vi "RunEcal.vi"(8 "error in (no error)":errorcluster, 11 "NetA_AgNA in":refnum<class "NetA_AgNA.lvclass">) -> (0 "error out":errorcluster {"code" format="%.0x"}, 2 "Error String":string, 3 "NetA_AgNA out":refnum<class "NetA_AgNA.lvclass">)   [LabVIEW 2014, in "NetA_AgNA.lvclass"]
doc: "Commands the eCal to make the specified measurements."
uses:
  NetA_AgNA.lvclass
  Tools/Station Calibration/RFSP MCT Calibration Tool/TypeDefs/TriggerMode_TypeDef.ctl
  Tools/Station Calibration/RFSP MCT Calibration Tool/TypeDefs/TriggerSource_TypeDef.ctl
  NetA_AgNA.lvclass/NetA_AgNA.ctl
  <instrlib>/Agilent NA/Agilent NA.lvlib
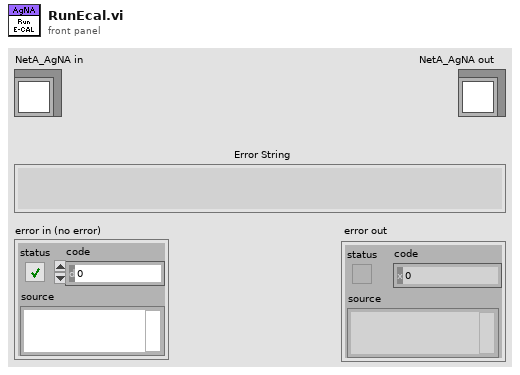
[diagram p1: front panel]
types:
  T1 = typedef "TriggerSource_TypeDef.ctl" = i32
  T2 = typedef "TriggerMode_TypeDef.ctl" = i32
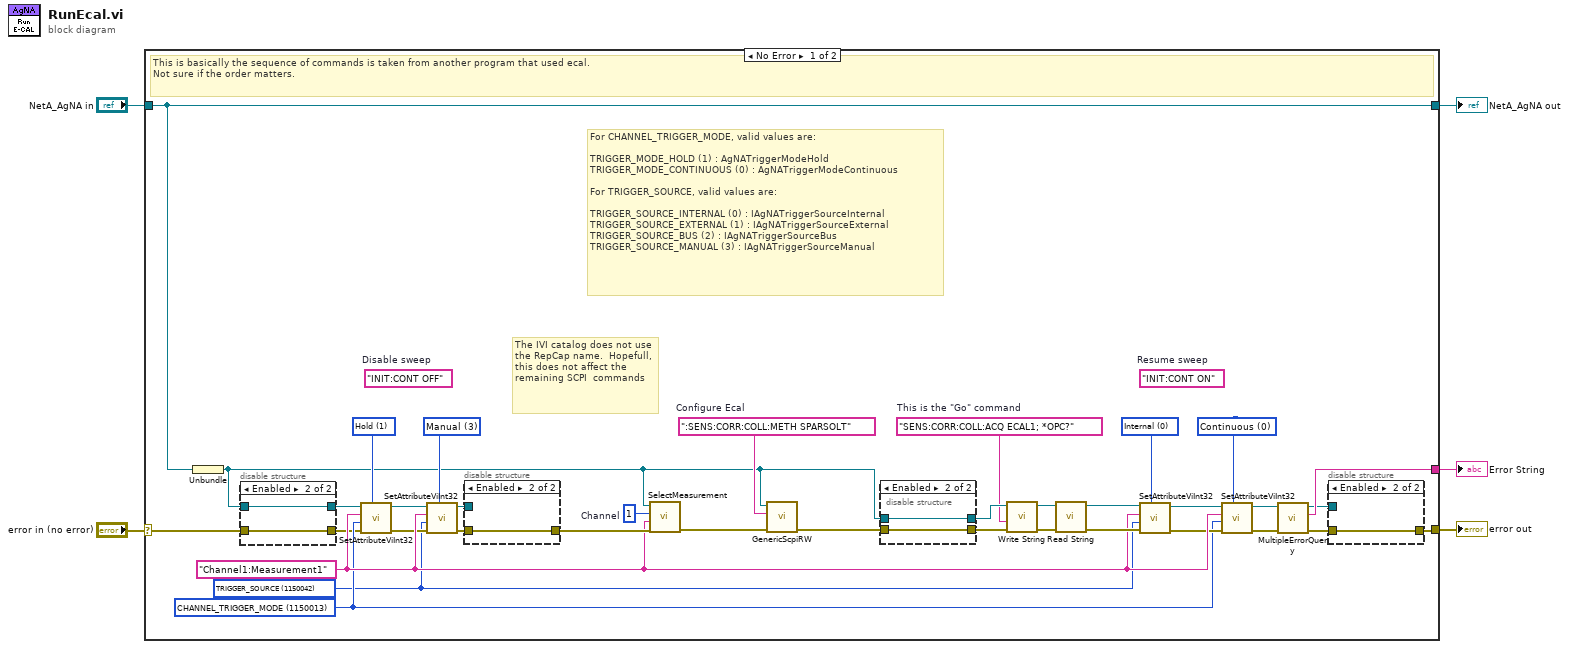
[diagram p0: block diagram]
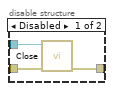
[diagram p2: hidden frame]
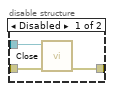
[diagram p3: hidden frame]
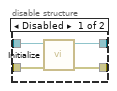
[diagram p4: hidden frame]
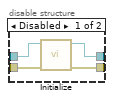
[diagram p5: hidden frame]
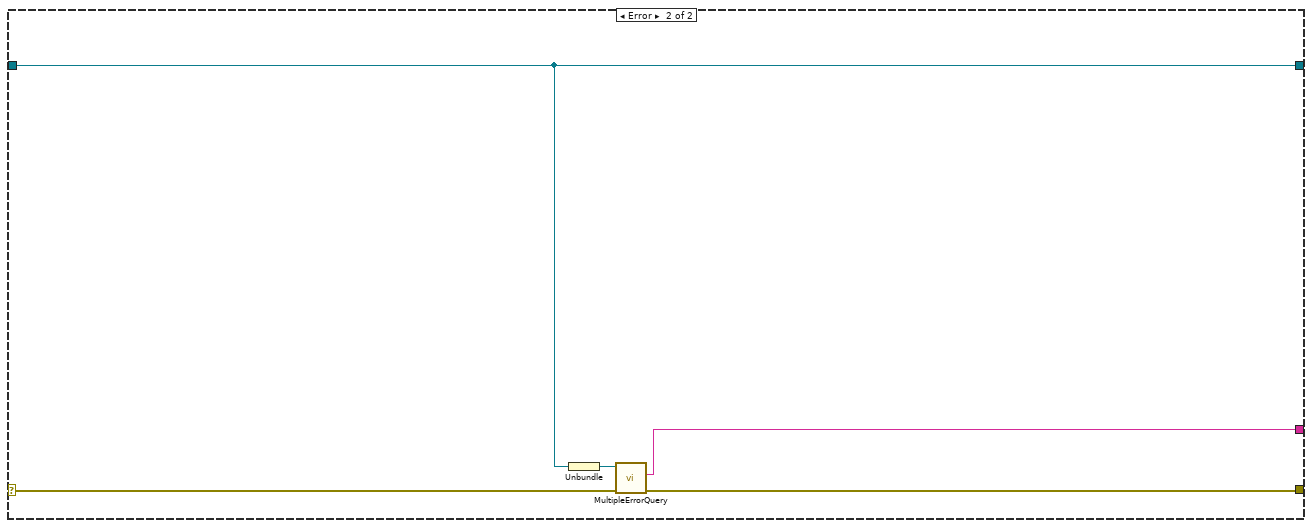
[diagram p6: hidden frame]
diagram:
  n1 = case shown="No Error" "error in (no error)" {
    selector: "error in (no error)" -> [w12 w66]
    tunnel: [w6 w65] -> w4
    tunnel: "NetA_AgNA in" -> [w14 w64]
    tunnel: [w14 w64] -> w2
    tunnel: [w15 w62] -> w1
    frame No Error {
      w13 = u32 1  # Channel
      w16 = T1 0 items=["Internal", "External", "Bus", "Manual"] ("Trigger Source Type")
      w17 = T1 3 items=["Internal", "External", "Bus", "Manual"] ("Trigger Source Type")
      w18 = T2 0 items=["Continuous", "Hold"] ("Trigger Mode Type")
      w19 = T2 1 items=["Continuous", "Hold"] ("Trigger Mode Type")
      (unwired) "INIT:CONT ON"  # Resume sweep
      (unwired) "INIT:CONT OFF"  # Disable sweep
      w23 = u32 1150013 items=["CHANNEL_AVERAGING_FACTOR"=1150002, "CHANNEL_MEASUREMENT_ELECTRICAL_DELAY_MEDIUM"=1150178, "CHANNEL_MEASUREMENT_ELECTRICAL_DELAY_UNITS"=1150175, "CHANNEL_MEASUREMENT_FORMAT"=1150014, "CHANNEL_MEASUREMENT_LIMIT_NUMBER"=1150020, "CHANNEL_MEASUREMENT_TIME_DOMAIN_GATING_SHAPE"=1150140, "CHANNEL_MEASUREMENT_TIME_DOMAIN_GATING_TYPE"=1150144, "CHANNEL_MEASUREMENT_TIME_DOMAIN_PARAMETERS"=1150137, "CHANNEL_MEASUREMENT_TIME_DOMAIN_TRANSFORM_MODE"=1150147, "CHANNEL_MEASUREMENT_TRACE_MATH"=1150017, "CHANNEL_POINTS"=1150007, "CHANNEL_SWEEP_MODE"=1150009, "CHANNEL_SWEEP_TYPE"=1150012, "CHANNEL_TRIGGER_MODE"=1150013, "DISPLAY_ARRANGE_WINDOWS"=1150181, "SYSTEM_TIME_OUT_MILLISECONDS"=1150040, "TRIGGER_SOURCE"=1150042, "WINDOW_SIZE"=1150133, "WINDOW_TABLE"=1150134] ("AttributeID")
      w22 = u32 1150042 items=["CHANNEL_AVERAGING_FACTOR"=1150002, "CHANNEL_MEASUREMENT_ELECTRICAL_DELAY_MEDIUM"=1150178, "CHANNEL_MEASUREMENT_ELECTRICAL_DELAY_UNITS"=1150175, "CHANNEL_MEASUREMENT_FORMAT"=1150014, "CHANNEL_MEASUREMENT_LIMIT_NUMBER"=1150020, "CHANNEL_MEASUREMENT_TIME_DOMAIN_GATING_SHAPE"=1150140, "CHANNEL_MEASUREMENT_TIME_DOMAIN_GATING_TYPE"=1150144, "CHANNEL_MEASUREMENT_TIME_DOMAIN_PARAMETERS"=1150137, "CHANNEL_MEASUREMENT_TIME_DOMAIN_TRANSFORM_MODE"=1150147, "CHANNEL_MEASUREMENT_TRACE_MATH"=1150017, "CHANNEL_POINTS"=1150007, "CHANNEL_SWEEP_MODE"=1150009, "CHANNEL_SWEEP_TYPE"=1150012, "CHANNEL_TRIGGER_MODE"=1150013, "DISPLAY_ARRANGE_WINDOWS"=1150181, "SYSTEM_TIME_OUT_MILLISECONDS"=1150040, "TRIGGER_SOURCE"=1150042, "WINDOW_SIZE"=1150133, "WINDOW_TABLE"=1150134] ("AttributeID")
      w30 = "Channel1:Measurement1" ("Meas Name")
      w36 = "SENS:CORR:COLL:ACQ ECAL1; *OPC?"  # This is the "Go" command
      w41 = ":SENS:CORR:COLL:METH SPARSOLT"  # Configure Ecal
      # "The IVI catalog does not use the RepCap name.  Hopefull, this does not affect the remaining SCPI  commands"
      # "For CHANNEL_TRIGGER_MODE, valid values are:\n\nTRIGGER_MODE_HOLD (1) : AgNATriggerModeHold\nTRIGGER_MODE_CONTINUOUS (0) : AgNATriggerModeContinuous\n\nFor TRIGGER_SOURCE, valid values are:\n\nTRIGGER_SOURCE_INTERNAL (0) : IAgNATriggerSourceInternal  \nTRIGGER_SOURCE_EXTERNAL (1) : IAgNATriggerSourceExternal\nTRIGGER_SOURCE_BUS (2) : IAgNATriggerSourceBus\nTRIGGER_SOURCE_MANUAL (3) : IAgNATriggerSourceManual"
      # "This is basically the sequence of commands is taken from another program that used ecal.\nNot sure if the order matters."
      n2 = Unbundle(w14) -> (w10:refnum<k15>)
      n3 = disable-structure shown="Enabled" {
        disable-tunnel: [w53 w55] -> w11
        disable-tunnel: [w52 w54] -> w9
        disable-tunnel: w12 -> [w51 w55]
        disable-tunnel: w10 -> [w50 w54]
        frame Disabled {
          n4 = call <instrlib>:"Initialize.vi"("error in (no error)"=w51, "resource name"=w50) -> ("error out"=w53:errorcluster, "instrument handle out"=w52:refnum<k15>)  [unwired: 8 in]
        }
        frame Enabled {
        }
      }
      n5 = call <instrlib>:"SetAttributeViInt32.vi"("AttributeValue"=w19, "error in (no error)"=w11, "AttributeID"=w23, "RepCapIdentifier"=w30, "instrument handle"=w9) -> ("error out"=w29:errorcluster, "instrument handle out"=w28:refnum<k15>)  [unwired: 5 in]
      n6 = call <instrlib>:"SetAttributeViInt32.vi"("AttributeValue"=w17, "error in (no error)"=w29, "AttributeID"=w22, "RepCapIdentifier"=w30, "instrument handle"=w28) -> ("error out"=w27:errorcluster, "instrument handle out"=w26:refnum<k15>)  [unwired: 5 in]
      n7 = disable-structure shown="Enabled" {
        disable-tunnel: [w48 w49] -> w33
        disable-tunnel: w27 -> [w47 w49]
        disable-tunnel: w26 -> [w46 _]
        frame Disabled {
          n8 = call <instrlib>:"Close.vi"("error in (no error)"=w47, "instrument handle"=w46) -> ("error out"=w48:errorcluster)  [unwired: 9 in]
        }
        frame Enabled {
        }
      }
      n9 = call "SelectMeasurement.vi"("error in (no error)"=w33, "Meas Name"=w30, "Channel"=w13, "resource name"=w10) -> ("error out"=w34:errorcluster)  [unwired: 7 in]
      n10 = call "GenericScpiRW.vi"("error in (no error)"=w34, "SCPI Command"=w41, "resource name"=w10) -> ("error out"=w35:errorcluster)  [unwired: 7 in, 1 out]
      n11 = disable-structure shown="Enabled" {
        disable-tunnel: [w59 w61] -> w40
        disable-tunnel: [w58 w60] -> w39
        disable-tunnel: w35 -> [w57 w61]
        disable-tunnel: w10 -> [w56 w60]
        frame Disabled {
          n12 = call <instrlib>:"Initialize.vi"("error in (no error)"=w57, "resource name"=w56) -> ("error out"=w59:errorcluster, "instrument handle out"=w58:refnum<k15>)  [unwired: 8 in]
        }
        frame Enabled {
        }
      }
      n13 = call <instrlib>:"Write String.vi"("error in (no error)"=w40, "Command"=w36, "instrument handle"=w39) -> ("error out"=w37:errorcluster, "instrument handle out"=w38:refnum<k15>)  [unwired: 7 in]
      n14 = call <instrlib>:"Read String.vi"("error in (no error)"=w37, "instrument handle"=w38) -> ("error out"=w32:errorcluster, "instrument handle out"=w31:refnum<k15>)  [unwired: 7 in, 1 out]
      n15 = call <instrlib>:"SetAttributeViInt32.vi"("AttributeValue"=w16, "error in (no error)"=w32, "AttributeID"=w22, "RepCapIdentifier"=w30, "instrument handle"=w31) -> ("error out"=w25:errorcluster, "instrument handle out"=w24:refnum<k15>)  [unwired: 5 in]
      n16 = call <instrlib>:"SetAttributeViInt32.vi"("AttributeValue"=w18, "error in (no error)"=w25, "AttributeID"=w23, "RepCapIdentifier"=w30, "instrument handle"=w24) -> ("error out"=w21:errorcluster, "instrument handle out"=w20:refnum<k15>)  [unwired: 5 in]
      n17 = call "MultipleErrorQuery.vi"("error in (no error)"=w21, "instrument handle"=w20) -> ("error out"=w8:errorcluster, "Error String"=w15:string, "instrument handle out"=w7:refnum<k15>)  [unwired: 7 in]
      n18 = disable-structure shown="Enabled" {
        disable-tunnel: [w44 w45] -> w6
        disable-tunnel: w8 -> [w43 w45]
        disable-tunnel: w7 -> [w42 _]
        frame Disabled {
          n19 = call <instrlib>:"Close.vi"("error in (no error)"=w43, "instrument handle"=w42) -> ("error out"=w44:errorcluster)  [unwired: 9 in]
        }
        frame Enabled {
        }
      }
    }
    frame Error {
      n20 = Unbundle(w64) -> (w63:refnum<k15>)
      n21 = call "MultipleErrorQuery.vi"("error in (no error)"=w66, "instrument handle"=w63) -> ("error out"=w65:errorcluster, "Error String"=w62:string)  [unwired: 7 in, 1 out]
    }
  }
  "error out" <- w4
  "NetA_AgNA out" <- w2
  "Error String" <- w1
